vi "position setpoint(SubVI)+7001.vi"(0 "Position 2":dbl=300.0, 1 "Position":dbl=300.0, 5 "Instrument Ref":refnum<k24>, 6 "队列输入":refnum<queue>, 7 "Delay":dbl, 9 "steps number":i32, 11 "Speed":i32=5 min=0 max=14, 12 "Resource In":refnum<visa-resource-name>, 15 "abort":refnum<queue>) -> (8 "错误输出":errorcluster)   [LabVIEW 2019, in "SubVI.lvlib"]
uses:
  SubVI.lvlib
  F:/ppms-6221&2182/QDInstrument_LabView (1)/QDInstrument.dll
  QDInstrument_LabView (1)/QDInstrument.dll
  Keithley 622x/Configure/Delta PDelta DCon Modes/Low Level/Typedefs/KE622x -- Delta PDelta Mode High Level.ctl
  KE7001.LLB/Keith 7001 Open/Close Chan.vi
  Keithley 622x/Keithley 622x.lvlib
panel:
  in  "通道":string
  in  "High Level In 1 (A)":T1=0.001 min=0.0 max=0.105 format="%.3p"
  in  "High Level In 2 (A)":T1=0.001 min=0.0 max=0.105 format="%.3p"
  out "数组":dbl[](array[numeric])
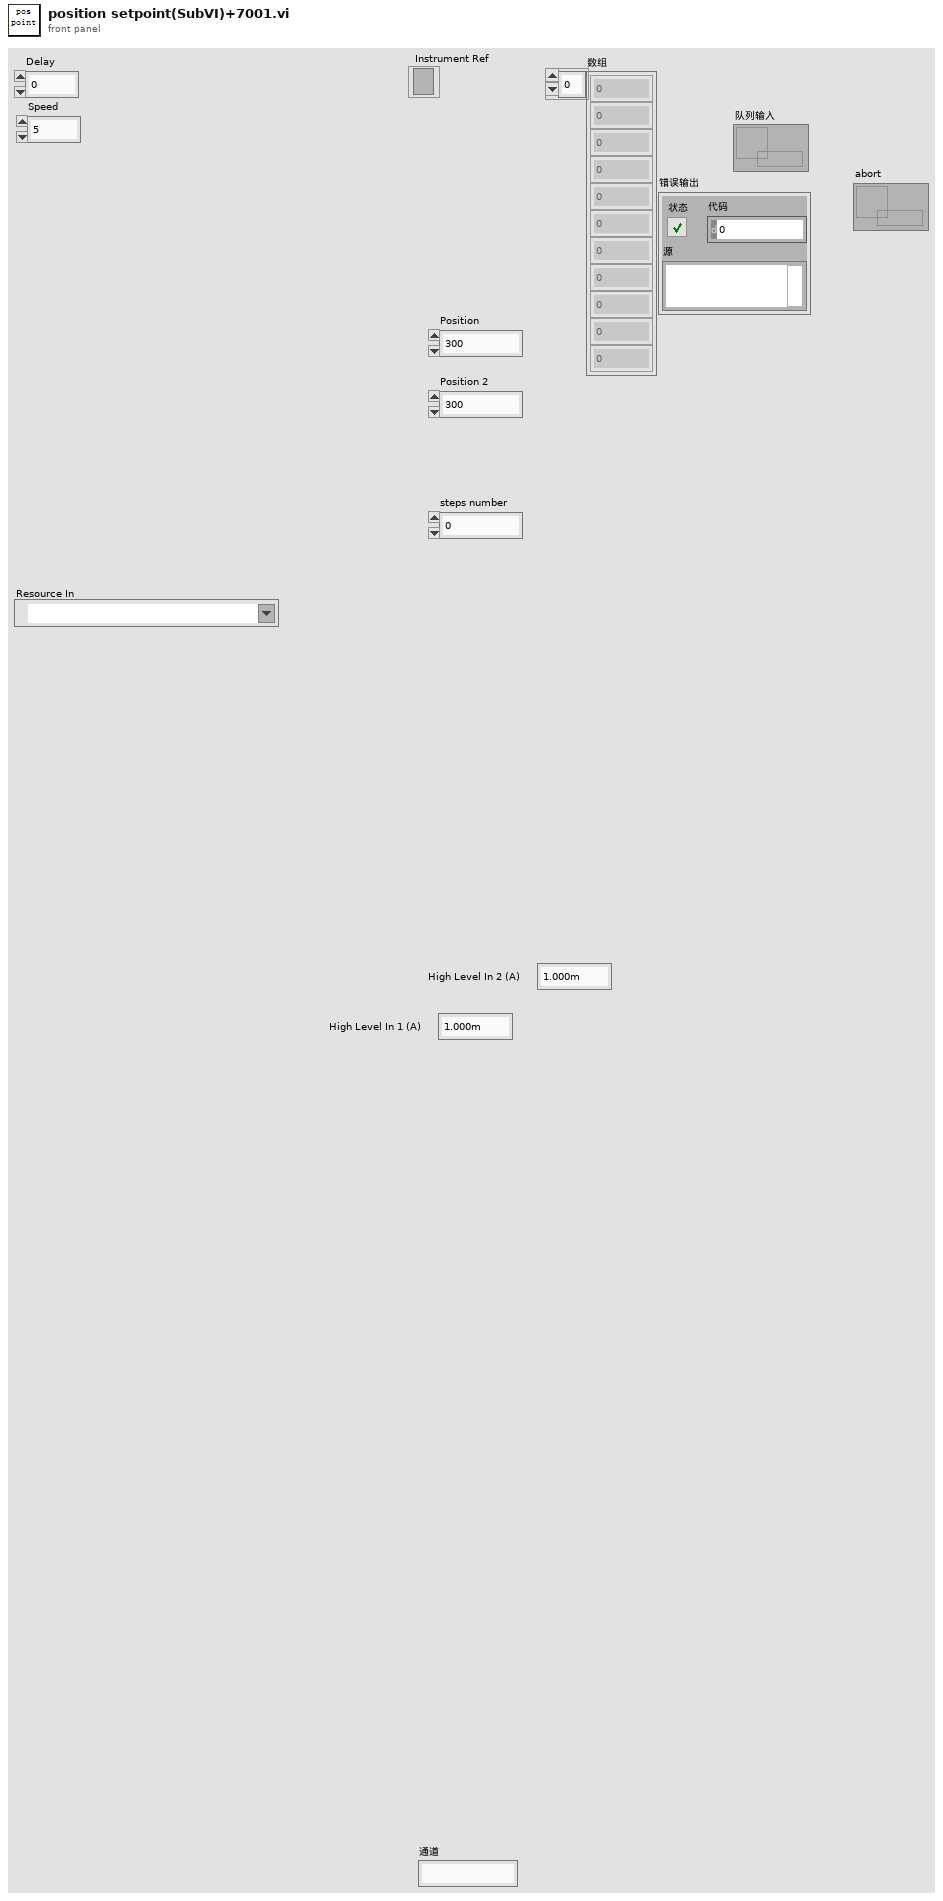
[diagram p1: front panel]
types:
  T1 = typedef "Keithley 622x.lvlib/KE622x -- Delta PDelta Mode High Level.ctl" = dbl
  T2 = cluster{"slot/memory":i16, "channel/row":i16, "column":i16, bool, bool}[]
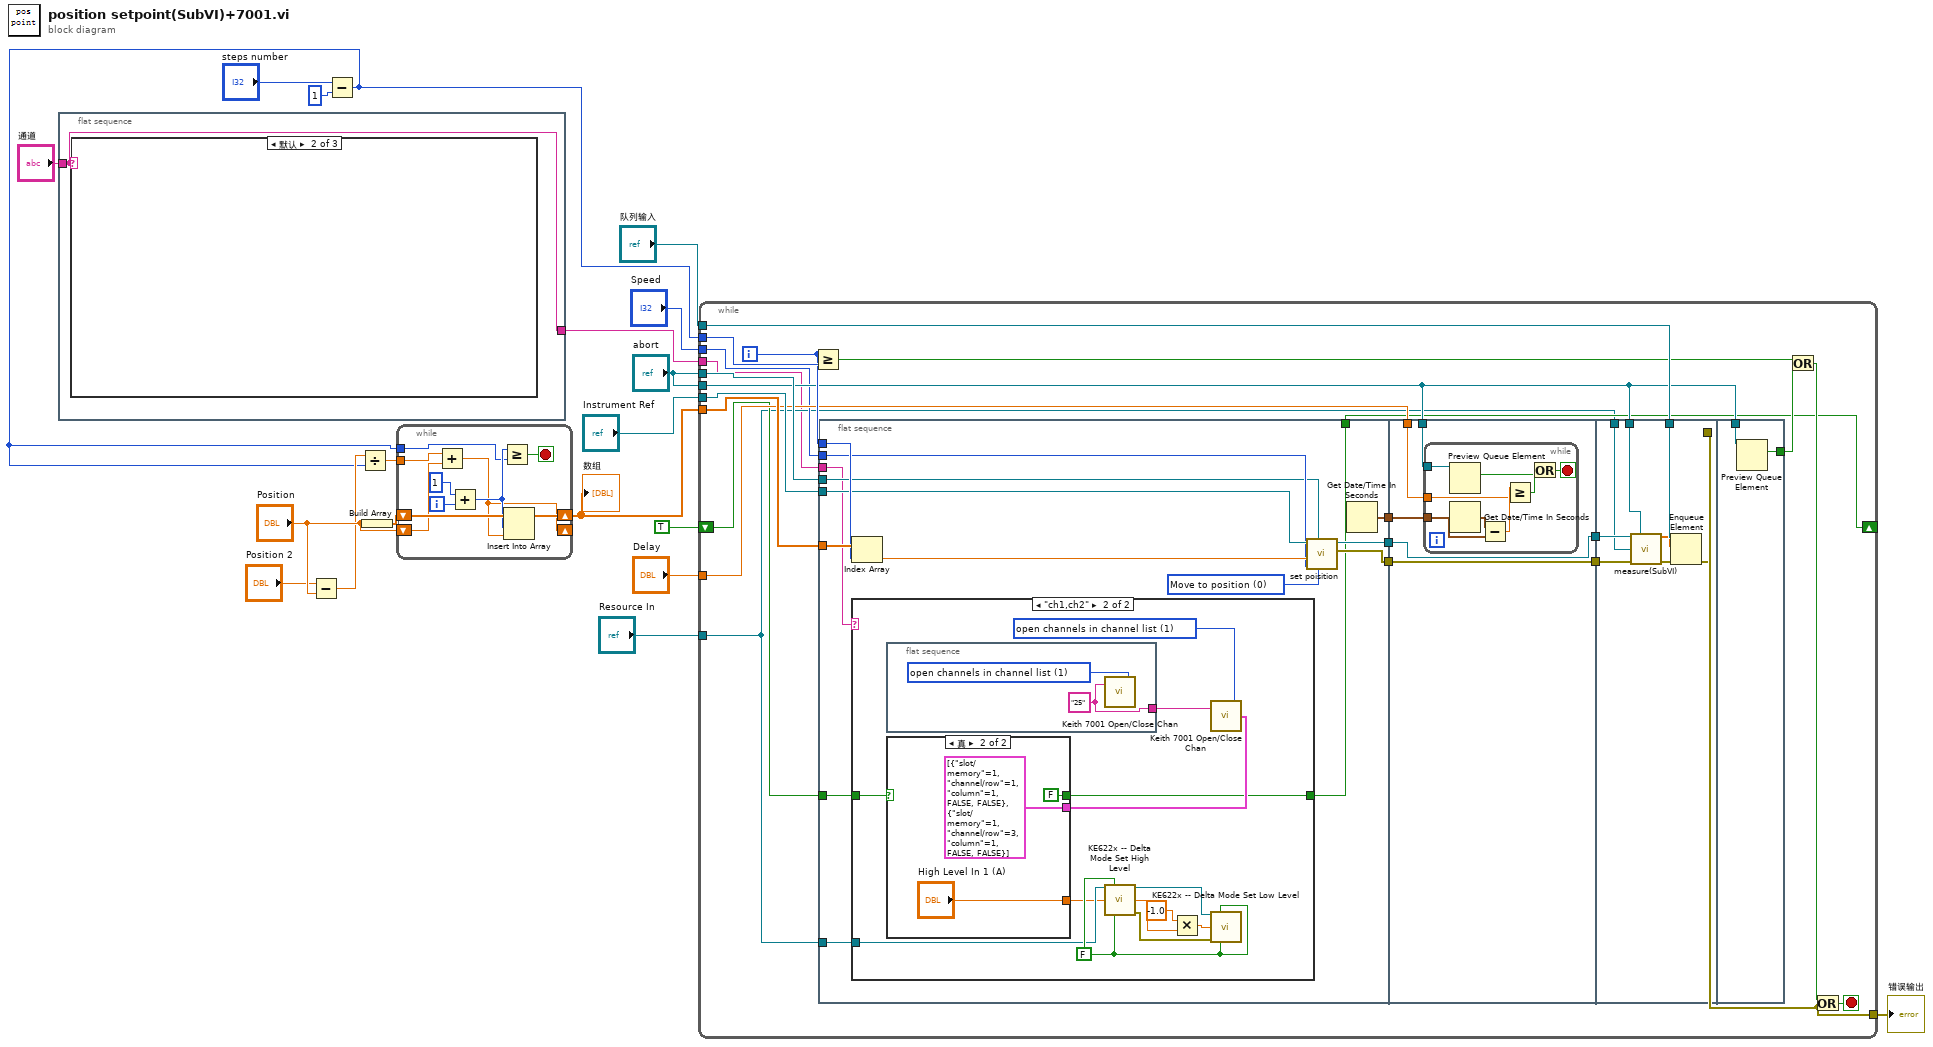
[diagram p0: block diagram]
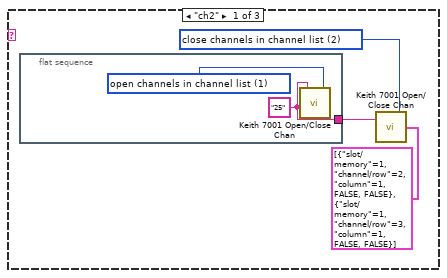
[diagram p2: hidden frame]
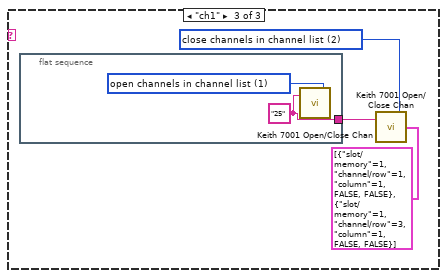
[diagram p3: hidden frame]
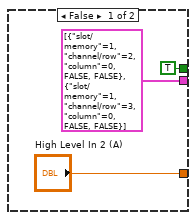
[diagram p5: hidden frame]
diagram:
  n1 = flat-sequence {
    tunnel: "通道" -> [w20]
    tunnel: [w20] -> w1
    frame #0 {
      n2 = case shown="默认" w20 {
        frame "ch2" {
          w22 = u16 2 items=["open all channels", "open channels in channel list", "close channels in channel list"] ("open/close (open all:0)")
          n3 = flat-sequence {
            tunnel: [w24] -> w23
            frame #0 {
              w25 = u16 1 items=["open all channels", "open channels in channel list", "close channels in channel list"] ("open/close (open all:0)")
              w24 = "25" ("GPIB address")
              n4 = call "Keith 7001 Open/Close Chan.vi"("GPIB address"=w24, "open/close (open all:0)"=w25) -> ()  [unwired: 2 in, 1 out]
            }
          }
          n5 = call "Keith 7001 Open/Close Chan.vi"("GPIB address"=w23, "open/close (open all:0)"=w22, "channel list"=T2 [{"slot/memory"=1, "channel/row"=2, "column"=1, FALSE, FALSE}, {"slot/memory"=1, "channel/row"=3, "column"=1, FALSE, FALSE}]) -> ()  [unwired: 1 in, 1 out]
        }
        frame Default {
        }
        frame "ch1" {
          w27 = u16 2 items=["open all channels", "open channels in channel list", "close channels in channel list"] ("open/close (open all:0)")
          n6 = flat-sequence {
            tunnel: [w29] -> w28
            frame #0 {
              w30 = u16 1 items=["open all channels", "open channels in channel list", "close channels in channel list"] ("open/close (open all:0)")
              w29 = "25" ("GPIB address")
              n7 = call "Keith 7001 Open/Close Chan.vi"("GPIB address"=w29, "open/close (open all:0)"=w30) -> ()  [unwired: 2 in, 1 out]
            }
          }
          n8 = call "Keith 7001 Open/Close Chan.vi"("GPIB address"=w28, "open/close (open all:0)"=w27, "channel list"=T2 [{"slot/memory"=1, "channel/row"=1, "column"=1, FALSE, FALSE}, {"slot/memory"=1, "channel/row"=3, "column"=1, FALSE, FALSE}]) -> ()  [unwired: 1 in, 1 out]
        }
      }
    }
  }
  n9 = Subtract(x="Position 2", y="Position") -> (x-y=w16:dbl)
  n10 = Subtract(x="steps number", y=1) -> (x-y=w7:i32)
  n11 = Divide(x=w16, y=w7) -> (x/y=w18:dbl)
  n12 = Build Array("Position") -> (w17:dbl[])
  n13 = while {
    shift-right: [w40] -> w14
    shift-left: w17 -> [w39]
    tunnel: w18 -> [w34]
    tunnel: w7 -> [w33]
    shift-right: [w32] -> _
    shift-left: "Position" -> [w31]
    i -> [w38]
    stop <- w35 stop-if-true
    n14 = Add(x=w34, y=w31) -> (x+y=w32:dbl)
    n15 = Add(x=1, y=w38) -> (x+y=w36:i32)
    n16 = Greater Or Equal?(x=w36, y=w33) -> (x >= y?=w35:bool)
    n17 = Insert Into Array(array=w39, index=w36, new element=w32) -> (w40:dbl[])
  }
  "数组" <- w14
  n18 = while {
    tunnel: w7 -> [w60]
    tunnel: "队列输入" -> [w63]
    tunnel: "abort" -> [w47]
    tunnel: "Instrument Ref" -> [w58]
    tunnel: w14 -> [w57]
    tunnel: "abort" -> [w56]
    tunnel: [w45] -> w10
    tunnel: "Delay" -> [w48]
    tunnel: "Speed" -> [w46]
    tunnel: "Resource In" -> [w42]
    shift-right: [w44] -> _
    shift-left: TRUE -> [w43]
    tunnel: w1 -> [w41]
    i -> [w59]
    stop <- w54 stop-if-true
    n19 = Greater Or Equal?(x=w59, y=w60) -> (x >= y?=w62:bool)
    n20 = flat-sequence {
      tunnel: [w68] -> w53
      tunnel: w59 -> [w75]
      tunnel: w58 -> [w74]
      tunnel: w57 -> [w76]
      tunnel: w56 -> [w69]
      tunnel: [w73] -> w51
      tunnel: [w72] -> w49
      tunnel: w46 -> [w71]
      tunnel: [w67] -> w44
      tunnel: w43 -> [w66]
      tunnel: w42 -> [w65]
      tunnel: w41 -> [w64]
      tunnel: w53 -> [w104]
      tunnel: [w104] -> w52
      tunnel: w51 -> [w103]
      tunnel: [w103] -> w50
      tunnel: w49 -> [w102]
      tunnel: w48 -> [w101]
      tunnel: w47 -> [w100]
      tunnel: w52 -> [w120]
      tunnel: w63 -> [w119]
      tunnel: [w113] -> w45
      tunnel: w47 -> [w117]
      tunnel: w50 -> [w116]
      tunnel: w42 -> [w115]
      tunnel: w47 -> [w122]
      tunnel: [w121] -> w61
      frame #0 {
        w70 = u16 0 items=["Move to position", "Move to limit", "Redefine current position"] ("Mode")
        n21 = Index Array(array=w76, index=w75) -> (element=w77:dbl)
        n22 = case shown="\"ch1,ch2\"" w64 {
          tunnel: [w78 w88] -> w67
          tunnel: w66 -> [w78 w87]
          tunnel: w65 -> [_ w80]
          frame "假", Default {
          }
          frame "ch1,ch2" {
            w81 = FALSE
            w91 = u16 1 items=["open all channels", "open channels in channel list", "close channels in channel list"] ("open/close (open all:0)")
            n23 = flat-sequence {
              tunnel: [w98] -> w90
              frame #0 {
                w99 = u16 1 items=["open all channels", "open channels in channel list", "close channels in channel list"] ("open/close (open all:0)")
                w98 = "25" ("GPIB address")
                n24 = call "Keith 7001 Open/Close Chan.vi"("GPIB address"=w98, "open/close (open all:0)"=w99) -> ()  [unwired: 2 in, 1 out]
              }
            }
            n25 = case shown="真" w87 {
              tunnel: [T2 [{"slot/memory"=1, "channel/row"=2, "column"=0, FALSE, FALSE}, {"slot/memory"=1, "channel/row"=3, "column"=0, FALSE, FALSE}] ("channel list") T2 [{"slot/memory"=1, "channel/row"=1, "column"=1, FALSE, FALSE}, {"slot/memory"=1, "channel/row"=3, "column"=1, FALSE, FALSE}] ("channel list")] -> w89
              tunnel: [TRUE FALSE] -> w88
              tunnel: ["High Level In 2 (A)" "High Level In 1 (A)"] -> w79
              frame False {
              }
              frame True {
              }
            }
            n26 = call "KE622x -- Delta Mode Set High Level.vi"("Resource In"=w80, "Check For SCPI Errors? (T)"=w81, "High Level In (A)"=w79, "Read Back Set Value? (T)"=w81) -> ("Resource Out (dupl)"=w86:refnum<visa-resource-name>, "High Level Out (A)"=w85:T1, "error out"=w82:errorcluster)  [unwired: 9 in]
            n27 = Multiply(x=T1 -1.0, y=w85) -> (x*y=w83:T1)
            n28 = call "Keith 7001 Open/Close Chan.vi"("GPIB address"=w90, "open/close (open all:0)"=w91, "channel list"=w89) -> ()  [unwired: 1 in, 1 out]
            n29 = call "KE622x -- Delta Mode Set Low Level.vi"("Resource In"=w86, "Check For SCPI Errors? (T)"=w81, "Low Level In (A)"=w83, "error in (no error)"=w82, "Read Back Set Value? (T)"=w81) -> ()  [unwired: 8 in, 3 out]
          }
        }
        n30 = call "set poisition.vi"("Mode"=w70, "abort"=w69, "Slow down code\ndefault = 0"=w71, "Position (deg)"=w77, "Instrument Ref In"=w74) -> ("error out"=w73:errorcluster, "Instrument Ref Out"=w68:refnum<k24>)  [unwired: 3 in]
        n31 = Get Date/Time In Seconds() -> (seconds since 1Jan1904=w72:timestamp)
      }
      frame #1 {
        n32 = while {
          tunnel: w102 -> [w111]
          tunnel: w101 -> [w109]
          tunnel: w100 -> [w107]
          stop <- w105 stop-if-true
          n33 = Preview Queue Element(queue=w107) -> (element=w106:bool)  [unwired: 2 in, 3 out]
          n34 = Get Date/Time In Seconds() -> (seconds since 1Jan1904=w112:timestamp)
          n35 = Subtract(x=w112, y=w111) -> (x-y=w110:dbl)
          n36 = Greater Or Equal?(x=w110, y=w109) -> (x >= y?=w108:bool)
          n37 = Or(x=w108, y=w106) -> (x .or. y?=w105:bool)
        }
      }
      frame #2 {
        n38 = call "measure(SubVI).vi"(".NET引用句柄输入"=w120, "error"=w117, "Resource In"=w115, "error in (no error)"=w116) -> ("data"=w118:dbl[], "error out"=w114:errorcluster)  [unwired: 10 in]
        n39 = Enqueue Element(queue=w119, element=w118, error in (no error)=w114) -> (error out=w113:errorcluster)  [unwired: 1 in, 2 out]
      }
      frame #3 {
        n40 = Preview Queue Element(queue=w122) -> (element=w121:bool)  [unwired: 2 in, 3 out]
      }
    }
    n41 = Or(x=w62, y=w61) -> (x .or. y?=w55:bool)
    n42 = Or(x=w55, y=w45) -> (x .or. y?=w54:bool)
  }
  "错误输出" <- w10
